vi "getItem.vi"(8 "error in (no error)":errorcluster caption="错误输入（无错误）", 10 "±í†Î”µ“þ":T1, 11 "HttpClient 输入":refnum<class "Http.lvclass"> caption="DNL_LabVIEW Object in") -> (0 "error out":errorcluster caption="错误输出", 2 "”µ“þ":string, 3 "HttpClient 输出":refnum<class "Http.lvclass"> caption="DNL_LabVIEW Object out")   [LabVIEW 2012, in "Http.lvclass"]
uses:
  Http.lvclass
  HttpData.ctl
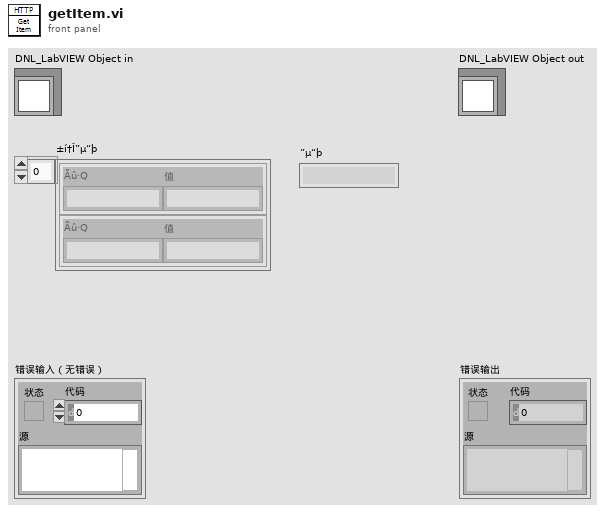
[diagram p1: front panel]
types:
  T1 = typedef "Http.lvclass/HttpData.ctl" = cluster{"Ãû·Q":string, "值":string}[]
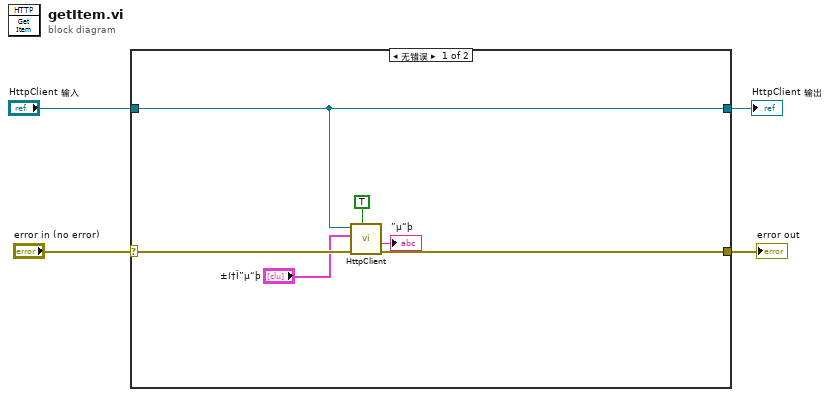
[diagram p0: block diagram]
diagram:
  n1 = case shown="无错误" "error in (no error)" {
    selector: "error in (no error)" -> [w10 w12]
    tunnel: [w9 w12] -> w3
    tunnel: [w8 w11] -> w1
    tunnel: "HttpClient 输入" -> [w8 w11]
    frame No Error {
      n2 = call-dynamic "HttpClient.vi"("™z²é î‘B?"=TRUE, "error in (no error)"=w10, "±í†Î”µ“þ"="±í†Î”µ“þ", "HttpClient 输入"=w8) -> ("error out"=w9:errorcluster, "”µ“þ"=→"”µ“þ":string)  [unwired: 2 in, 4 out]
    }
    frame Error {
    }
  }
  "error out" <- w3
  "HttpClient 输出" <- w1
